vi "interpolate.vi"(8 "error in (no error)":errorcluster, 10 "Power in":dbl, 11 "AOTF in":refnum<class "AOTF.lvclass">) -> (0 "error out":errorcluster, 2 "Power voltage out":dbl, 3 "AOTF out":refnum<class "AOTF.lvclass">)   [LabVIEW 2012, in "AOTF.lvclass"]
uses:
  AOTF.lvclass
  AOTF.lvclass/AOTF.ctl
  <vilib>/gmath/NI_Gmath.lvlib
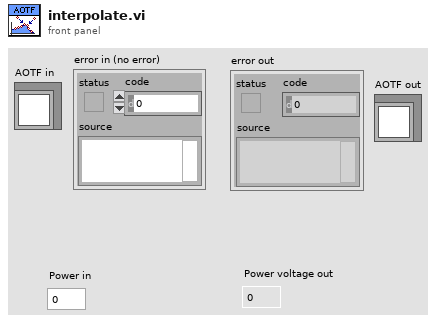
[diagram p1: front panel]
types:
  T1 = typedef "AOTF.lvclass/laser line ring.ctl" = u8
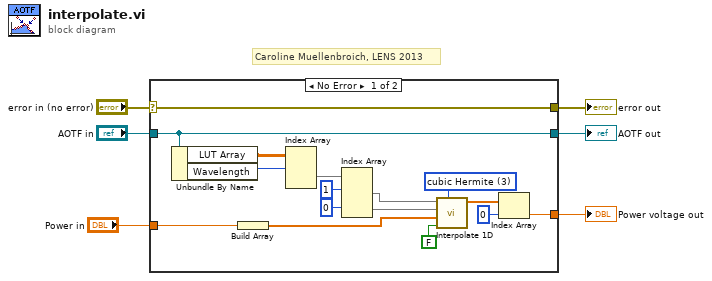
[diagram p0: block diagram]
diagram:
  # "Caroline Muellenbroich, LENS 2013"
  n1 = case shown="No Error" "error in (no error)" {
    selector: "error in (no error)" -> [w22 w24]
    tunnel: [w22 w24] -> w5
    tunnel: [w19 w23] -> w4
    tunnel: "AOTF in" -> [w19 w23]
    tunnel: "Power in" -> [w16 _]
    tunnel: [w9 _] -> w1
    frame No Error {
      w21 = 3 items=["nearest", "linear", "spline", "cubic Hermite", "Lagrange"] ("method")
      n2 = Unbundle By Name(w19) -> ("LUT Array"=w18:dbl[][][], "Wavelength"=w17:T1)
      n3 = Build Array(w16) -> (w12:dbl[])
      n4 = Index Array(array=w18, index (dim 0)=w17) -> (element=w15:dbl[][])  [unwired: 2 in]
      n5 = Index Array(array=w15, index (row) #1=1 ("index (row)"), index (row) #2=0 ("index (row)")) -> (element #1=w14:dbl[], element #2=w13:dbl[])  [unwired: 2 in]
      n6 = call <vilib>:"Interpolate 1D.vi"("method"=w21, "X is monotonic"=FALSE, "xi"=w12, "X"=w13, "Y"=w14) -> ("yi"=w10:dbl[])  [unwired: 4 in, 2 out]
      n7 = Index Array(array=w10, index=0) -> (element=w9:dbl)
    }
    frame Error {
    }
  }
  "error out" <- w5
  "AOTF out" <- w4
  "Power voltage out" <- w1
